vi "Event.vi"() -> ()   [LabVIEW 2023]
panel:
  in  "Stop Button":bool
  in  "c":bool
  in  "b":bool
  in  "a":bool
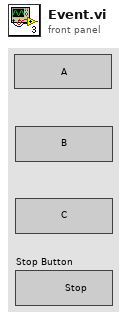
[diagram p1: front panel]
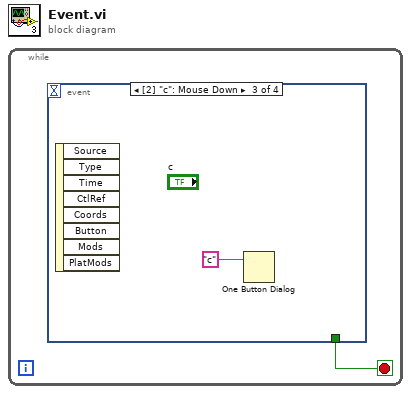
[diagram p0: block diagram]
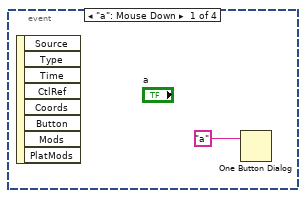
[diagram p2: hidden frame]
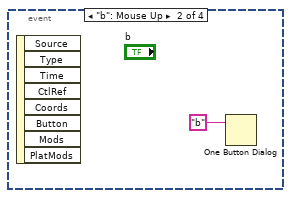
[diagram p3: hidden frame]
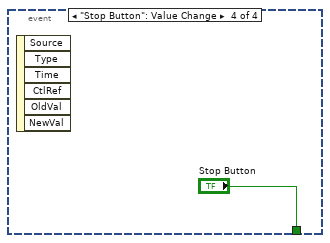
[diagram p4: hidden frame]
diagram:
  n1 = while {
    stop <- w1 stop-if-true
    n2 = event shown="[2] \"c\": Mouse Down" {
      selector: _ -> [_ _ _ _]
      dyn-events: _ -> [_ _ _ _]
      timeout: _ -> [_ _ _ _]
      tunnel: [_ _ _ "Stop Button"] -> w1
      event "a": Mouse Down {
        n3 = event-data() -> ()  [unwired: 1 in, 8 out]
        n4 = One Button Dialog(message="a") -> ()  [unwired: 1 in, 1 out]
      }
      event "b": Mouse Up {
        n5 = event-data() -> ()  [unwired: 1 in, 8 out]
        n6 = One Button Dialog(message="b") -> ()  [unwired: 1 in, 1 out]
      }
      event "c": Mouse Down {
        n7 = event-data() -> ()  [unwired: 1 in, 8 out]
        n8 = One Button Dialog(message="c") -> ()  [unwired: 1 in, 1 out]
      }
      event "Stop Button": Value Change {
        n9 = event-data() -> ()  [unwired: 1 in, 6 out]
      }
    }
  }
